vi "Write XY graph ref.vi"(8 "error in (no error)":errorcluster, 9 "Combo Box":string(combo)="Kinetics", 10 "XY graph ref":refnum<vi>, 11 "Control-Client in":refnum<class "Control-Client.lvclass">) -> (0 "error out":errorcluster, 3 "Control-Client out":refnum<class "Control-Client.lvclass">)   [LabVIEW 2019, in "Control-Client.lvclass"]
uses:
  Control-Client.lvclass
  Control-Client.lvclass/Control-Client.ctl
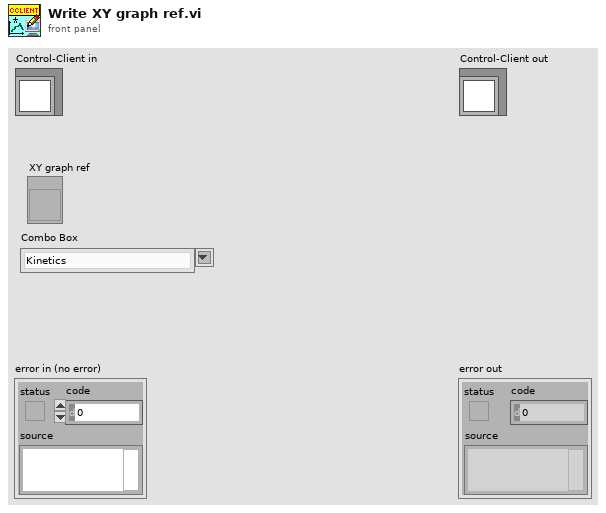
[diagram p1: front panel]
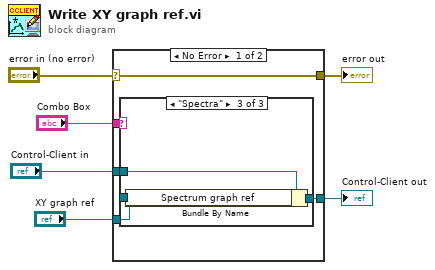
[diagram p0: block diagram]
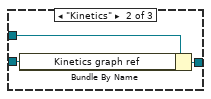
[diagram p3: hidden frame]
diagram:
  n1 = case shown="No Error" "error in (no error)" {
    selector: "error in (no error)" -> [w11 w19]
    tunnel: [w11 w19] -> w5
    tunnel: [w9 w20] -> w3
    tunnel: "Control-Client in" -> [w10 w20]
    tunnel: "XY graph ref" -> [w8 _]
    tunnel: "Combo Box" -> [w7 _]
    frame No Error {
      n2 = case shown="\"Spectra\"" w7 {
        tunnel: w10 -> [w12 w15 w18]
        tunnel: [w12 w13 w17] -> w9
        tunnel: w8 -> [_ w14 w16]
        frame "False", Default {
        }
        frame "Kinetics" {
          n3 = Bundle By Name(cluster=w15, "Kinetics graph ref"=w14) -> (w13:refnum<class "Control-Client.lvclass">)
        }
        frame "Spectra" {
          n4 = Bundle By Name(cluster=w18, "Spectrum graph ref"=w16) -> (w17:refnum<class "Control-Client.lvclass">)
        }
      }
    }
    frame Error {
    }
  }
  "error out" <- w5
  "Control-Client out" <- w3
